vi "Mock Process Error On Request.vi"(8 "error in (no error)":errorcluster, 10 "Mock Error":errorcluster, 11 "Mock Process in":refnum<class "Mock Process.lvclass">) -> (0 "error out":errorcluster, 3 "Mock Process out":refnum<class "Mock Process.lvclass">)   [LabVIEW 2020, in "Mock Process.lvclass"]
uses:
  Mock Process.lvclass
  C:/Git/astemes-triarc-framework/source/Framework/Process/Process.lvclass
  Framework/Process/Process.lvclass/Process.ctl
  Framework/Process/Public/Lifecycle/Get Lifecycle State.vi
  Framework/Process/Private/SubVIs/Handle Debug Data.vi
  Framework/Process/Private/SubVIs/Enqueue Request Message.vi
  <vilib>/Utility/error.llb/Clear Errors.vi
  Framework/Logging/Log Debug.vi
  <vilib>/AdvancedString/1D String Array to Delimited String.vi
  <vilib>/Utility/High Resolution Relative Seconds.vi
  <vilib>/Utility/error.llb/Error Cluster From Error Code.vi
  Framework/Process/Public/Read Name.vi
  Framework/Process/Private/SubVIs/Wait for Response Message.vi
  Framework/Process/Process.lvclass
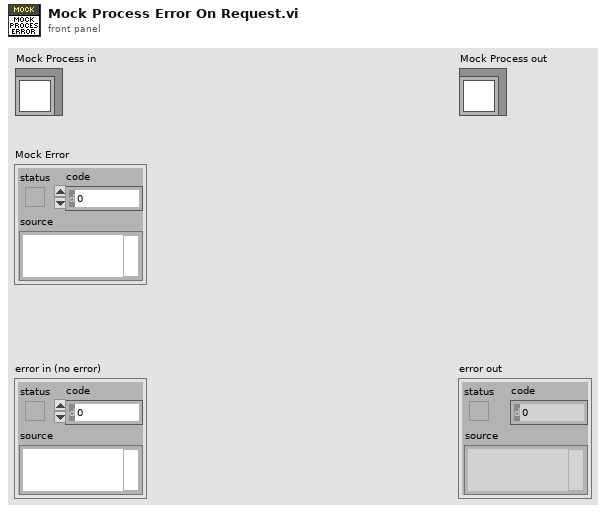
[diagram p1: front panel]
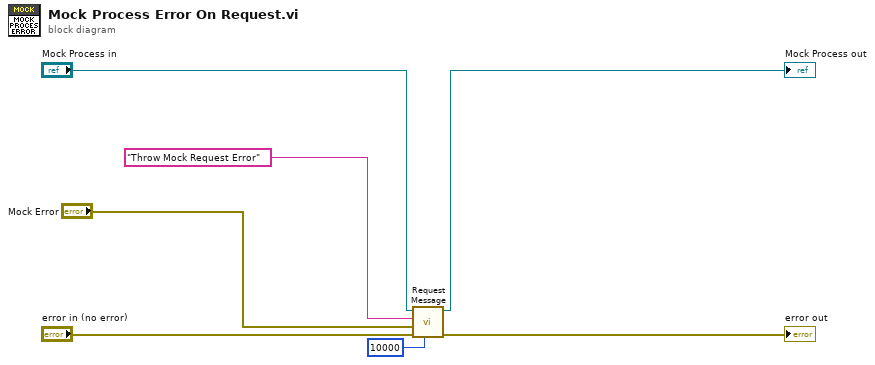
[diagram p0: block diagram]
diagram:
  n1 = call "Request Message.vi"("timeout in ms (-1)"=10000, "error in (no error)"="error in (no error)", "Request Message Data"="Mock Error", "Request Message"="Throw Mock Request Error", "Process In"="Mock Process in") -> ("error out"=→"error out":errorcluster, "Process Out"=→"Mock Process out":refnum<class "Mock Process.lvclass">)  [unwired: 2 in, 3 out]
